vi "Operate.vi"(8 "Error_In":errorcluster, 11 "Calculator_In":refnum<class "Calculator.lvclass">) -> (0 "Error_Out":errorcluster, 3 "Calculator_Out":refnum<class "Calculator.lvclass">)   [LabVIEW 2023, in "Calculator.lvclass"]
doc: "Used to do math operation by over riding"
uses:
  Calculator.lvclass
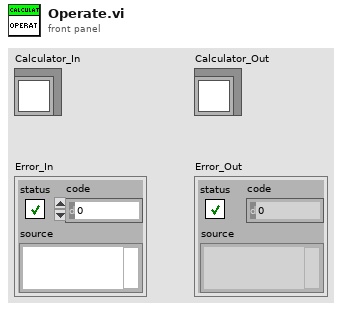
[diagram p1: front panel]
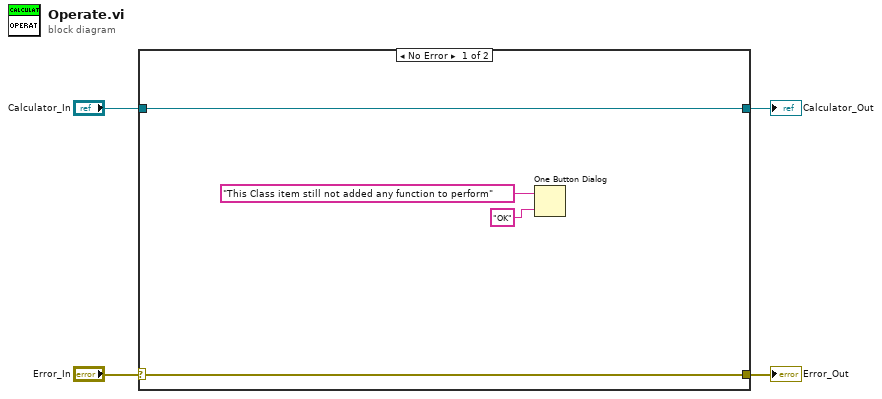
[diagram p0: block diagram]
diagram:
  n1 = case shown="No Error" "Error_In" {
    selector: "Error_In" -> [w7 w10]
    tunnel: [w7 w10] -> w3
    tunnel: [w8 w9] -> w1
    tunnel: "Calculator_In" -> [w8 w9]
    frame No Error {
      n2 = One Button Dialog(message="This Class item still not added any function to perform", button name ("OK")="OK") -> ()  [unwired: 1 out]
    }
    frame Error {
    }
  }
  "Error_Out" <- w3
  "Calculator_Out" <- w1
